vi "Calibration.vi"(7 "Load calibration data":bool, 8 "error in (no error)":errorcluster, 9 "Save calibration data":bool, 10 "Done Button":bool, 11 "Distance [cm]| Voltage [V]":dbl[][](array[numeric])) -> (0 "error out":errorcluster, 2 "Interpolation method":T1(ring), 3 "Distance [cm]| Voltage [V]":dbl[][](array[numeric]))   [LabVIEW 2022 SP3]
uses:
  <vilib>/Utility/file.llb/Write Delimited Spreadsheet (DBL).vi
  <vilib>/Utility/file.llb/Read Delimited Spreadsheet (DBL).vi
  <vilib>/gmath/NI_Gmath.lvlib
panel:
  in  "method":T1(ring)=enum."linear"
  in  "Refresh Button":bool
  out "Transfer function":cluster{"yi":dbl[], "xi used":dbl[]}[](graph)
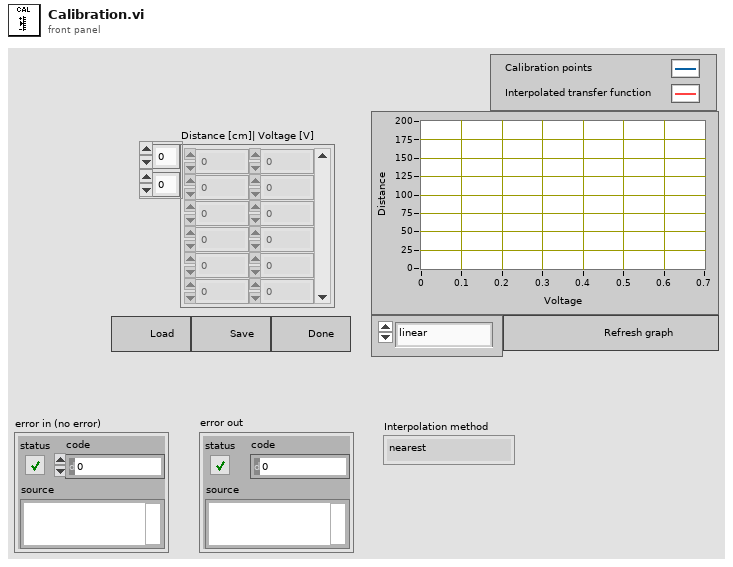
[diagram p1: front panel]
types:
  T1 = enum16{"nearest", "linear", "spline", "cubic Hermite", "Lagrange"}
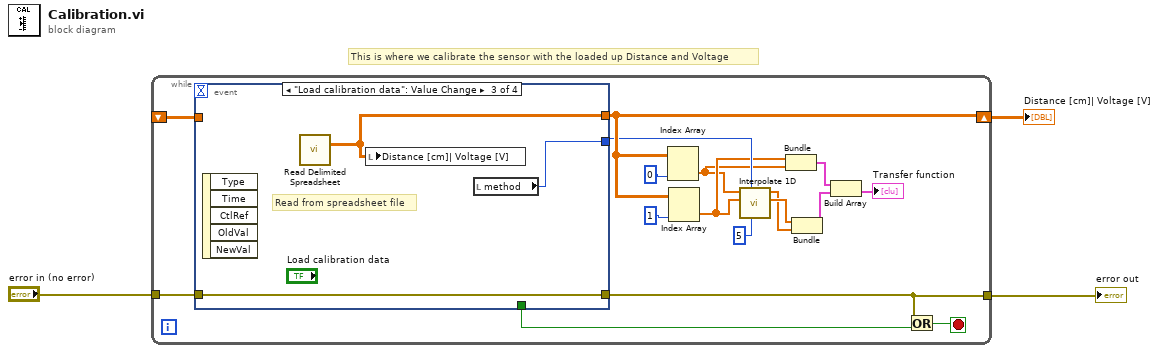
[diagram p0: block diagram]
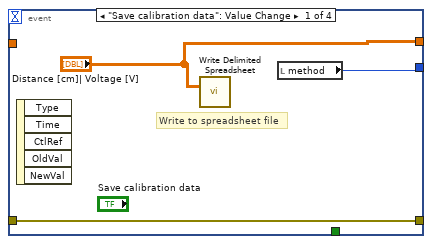
[diagram p2: hidden frame]
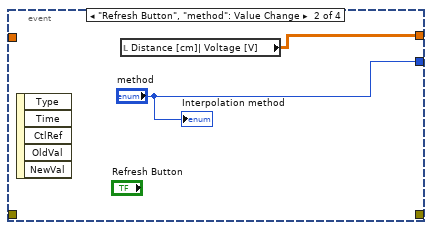
[diagram p3: hidden frame]
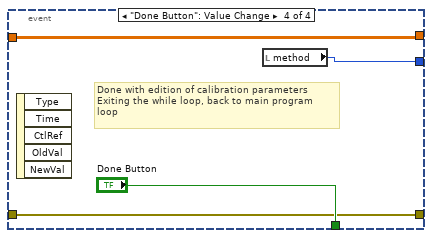
[diagram p4: hidden frame]
diagram:
  # "This is where we calibrate the sensor with the loaded up Distance and Voltage"
  n1 = while {
    tunnel: "error in (no error)" -> [w19]
    tunnel: [w18] -> w3
    shift-right: [w13] -> w1
    shift-left: _ -> [w20]
    stop <- w16 stop-if-true
    n2 = event shown="[2] \"Load calibration data\": Value Change" {
      selector: _ -> [_ _ _ _]
      dyn-events: _ -> [_ _ _ _]
      timeout: _ -> [_ _ _ _]
      tunnel: w20 -> [_ _ _ w32]
      tunnel: ["Distance [cm]| Voltage [V]" w25 w26 w32] -> w13
      tunnel: [_ _ _ "Done Button"] -> w17
      tunnel: w19 -> [w23 _ w28 w30]
      tunnel: [w23 _ w28 w30] -> w18
      tunnel: [w22 "method" w27 w29] -> w8
      event "Save calibration data": Value Change {
        # "Write to spreadsheet file"
        n3 = event-data() -> ()  [unwired: 1 in, 5 out]
        n4 = call-poly <vilib>:"Write Delimited Spreadsheet.vi"("2D data"="Distance [cm]| Voltage [V]") -> ()  [unwired: 13 in, 2 out]
        n5 = local read "method"() -> (w22:T1)
      }
      event "Refresh Button", "method": Value Change {
        n6 = event-data() -> ()  [unwired: 1 in, 5 out]
        n7 = local read "Distance [cm]| Voltage [V]"() -> (w25:dbl[][])
        "Interpolation method" <- "method"
      }
      event "Load calibration data": Value Change {
        # "Read from spreadsheet file"
        n8 = event-data() -> ()  [unwired: 1 in, 5 out]
        n9 = call-poly <vilib>:"Read Delimited Spreadsheet.vi"() -> ("all rows"=w26:dbl[][])  [unwired: 10 in, 5 out]
        n10 = local write "Distance [cm]| Voltage [V]"(w26) -> ()
        n11 = local read "method"() -> (w27:T1)
      }
      event "Done Button": Value Change {
        # "Done with edition of calibration parameters\nExiting the while loop, back to main program \nloop"
        n12 = event-data() -> ()  [unwired: 1 in, 5 out]
        n13 = local read "method"() -> (w29:T1)
      }
    }
    n14 = Index Array(array=w13, index (col)=0 ("disabled index (col)")) -> (element=w6:dbl[])  [unwired: 1 in]
    n15 = Index Array(array=w13, index (col)=1 ("disabled index (col)")) -> (element=w7:dbl[])  [unwired: 1 in]
    n16 = call <vilib>:"Interpolate 1D.vi"("ntimes"=5, "method"=w8, "X"=w7, "Y"=w6) -> ("xi used"=w5:dbl[], "yi"=w4:dbl[])  [unwired: 5 in, 1 out]
    n17 = Bundle("all rows"=w7, "all rows"=w6) -> (w11:cluster{"all rows":dbl[], "all rows":dbl[]})  [unwired: 1 in]
    n18 = Bundle("xi used"=w5, "yi"=w4) -> (w10:cluster{"xi used":dbl[], "yi":dbl[]})  [unwired: 1 in]
    n19 = Build Array(w11, w10) -> (→"Transfer function":cluster{"xi used":dbl[], "yi":dbl[]}[])
    n20 = Or(x=w18, y=w17) -> (x .or. y?=w16:bool)
  }
  "error out" <- w3
  "Distance [cm]| Voltage [V]" <- w1
